vi "c_EnumToLvEnum.vi"() -> ()   [LabVIEW 2023]
uses:
  controls/motionStateMachineEnum.ctl
  <vilib>/Utility/error.llb/Trim Whitespace One-Sided.vi
panel:
  out "array":string[](array[string])
  in  "C enum":string
  in  "stateMachine":T1 items=["STATE_INIT", "STATE_FORWARD", "STATE_SLOW_FORWARD", "STATE_BACKWARD", "STATE_START_ROTATION", "STATE_ROTATION", "STATE_STOP", "STATE_DISTANCE", "STATE_WIRE", "STATE_HOME", "STATE_CHARGE", ""]
  # "enum stateMachine\n{\n\tSTATE_INIT,\n\tSTATE_FORWARD,\n\tSTATE_SLOW_FORWARD,\n\tSTATE_BACKWARD,\n\tSTATE_START_ROTATION,\n\tSTATE_ROTATION,\n\tSTATE_STOP,\n\tSTATE_DISTANCE,\n\tSTATE_WIRE,\n\tSTATE_HOME,\n\tSTATE_CHARGE,\n\tSTATE_ERROR\n};"
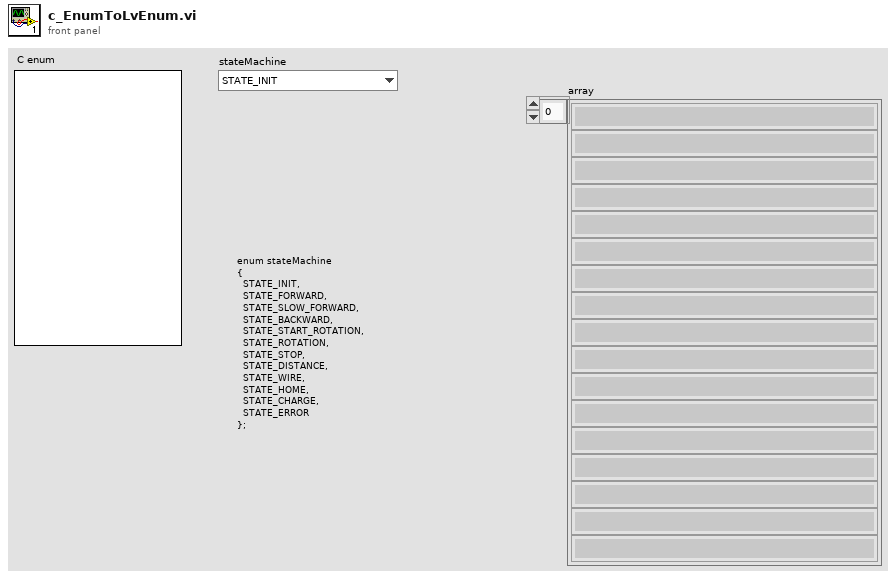
[diagram p1: front panel]
types:
  T1 = typedef "motionStateMachineEnum.ctl" = u16
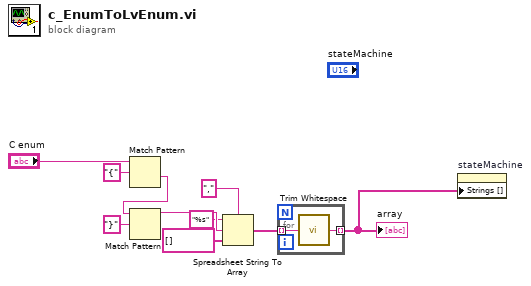
[diagram p0: block diagram]
diagram:
  n1 = Match Pattern(string="C enum", regular expression="{") -> (after substring=w7:string)  [unwired: 1 in, 3 out]
  n2 = Match Pattern(string=w7, regular expression="}") -> (before substring=w6:string)  [unwired: 1 in, 3 out]
  n3 = Spreadsheet String To Array(delimiter (Tab)=",", format string="%s", spreadsheet string=w6, array type (2D Dbl)=string[] []) -> (array=w2:string[])
  n4 = for {
    tunnel: w2 -> [w12] mode=indexing
    tunnel: [w11] -> w1 mode=indexing
    n5 = call <vilib>:"Trim Whitespace.vi"("string"=w12) -> ("trimmed string"=w11:string)  [unwired: 1 in]
  }
  "array" <- w1
  n6 = property on="stateMachine" class="Ring (strict)"("Strings []"=w1) -> ()  [unwired: 2 in, 2 out]
